vi "MercuryIPSWait.vi"(0 "Inst_param":T3={"Kind"=0, "Strings"=["", "192.168.137.3", "T", "GRPZ"], "uint64s"=[], "Doubles"=[-12.0, 12.0, 6.285], "DAQmx take out list"=[]}) -> ()   [LabVIEW 2013]
uses:
  <instrlib>/Mercury iXX/Public/Controls/Comms Transport Layer.ctl
  <instrlib>/Mercury iXX/Public/Controls/Serial Settings.ctl
  <instrlib>/Mercury iXX/Public/Controls/ISOBus Address.ctl
  <instrlib>/Mercury iXX/Mercury iXX.lvlib
panel:
  out "Mag_data":T1
  out "Device Details":T2={"Devices"=["DB3.L1:LVL", "GRPS:PSU", "GRPX:PSU", "GRPY:PSU", "GRPZ:PSU", "MB1.T1:TEMP", "PSU.M1:PSU", "PSU.M2:PSU"], "S/W Version(s)"=[], "Serial Number(s)"=[]}
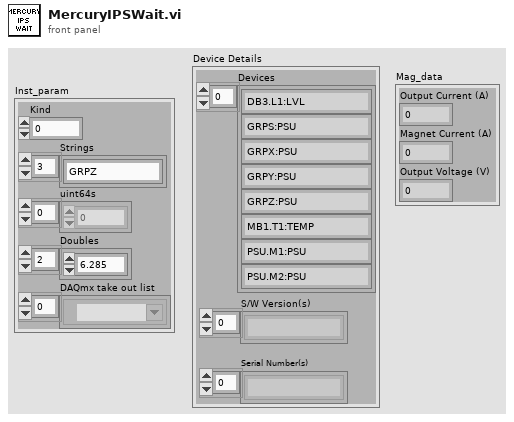
[diagram p1: front panel]
types:
  T1 = cluster{"Output Current (A)":dbl, "Magnet Current (A)":dbl, "Output Voltage (V)":dbl}
  T2 = cluster{"Devices":string[], "S/W Version(s)":string[], "Serial Number(s)":string[]}
  T3 = cluster{"Kind":u16, "Strings":string[], "uint64s":u64[], "Doubles":dbl[], "DAQmx take out list":refnum<k21>[]}
  T4 = typedef "Mercury iXX.lvlib/Comms Transport Layer.ctl" = enum16{"Ethernet TCP/IP", "USB", "ISOBus - RS-232", "GPIB"}
  T5 = typedef "Mercury iXX.lvlib/Serial Settings.ctl" = cluster{"Baud Rate":u32, "Parity":u16, "Data Bits":u16, "Stop Bits":u16, "Flow Control":u16}
  T6 = typedef "Mercury iXX.lvlib/ISOBus Address.ctl" = i32
  T7 = cluster{"VISA resource name":refnum<visa-resource-name>, "Comms Layer":T4, "IP Address":string, "Serial Configuration":T5, "ISOBUS address":T6}
  T8 = typedef "Mercury iXX.lvlib/Mercury Reference.ctl" = cluster{"Comms":refnum<visa-resource-name>, "Device ID":string[], "Comms Layer":T4, "Command":string, "Query reference":T9}
  T9 = typedef "Mercury iXX.lvlib/Query Dynamic Reference.ctl" = refnum<vi>
  T10 = enum16{"Monitor", "Hold", "Clamp", "To Set", "To Zero", "Switch Heater", "Set Points"}
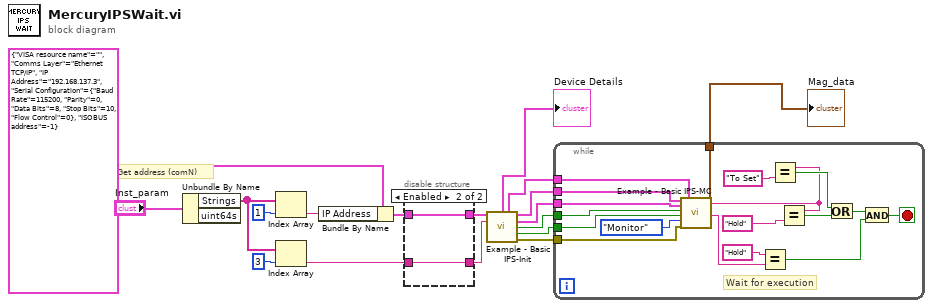
[diagram p0: block diagram]
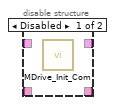
[diagram p2: hidden frame]
diagram:
  # "Get address (comN)"
  n1 = Unbundle By Name("Inst_param") -> ("Strings"=w4:string[])  [unwired: 1 out]
  n2 = Index Array(array=w4, index=1) -> (element=w17:string)
  n3 = Index Array(array=w4, index=3) -> (element=w2:string)
  n4 = Bundle By Name(cluster=T7 {"VISA resource name"="", "Comms Layer"=enum."Ethernet TCP/IP", "IP Address"="192.168.137.3", "Serial Configuration"={"Baud Rate"=115200, "Parity"=0, "Data Bits"=8, "Stop Bits"=10, "Flow Control"=0}, "ISOBUS address"=-1} ("Connection Details"), "IP Address"=w17) -> (w15:T7)
  n5 = disable-structure shown="Enabled" {
    disable-tunnel: [_ w20] -> w13
    disable-tunnel: w15 -> [_ w20]
    disable-tunnel: [_ w19] -> w3
    disable-tunnel: w2 -> [_ w19]
    frame Disabled {
      n6 = call "MDrive_Init_Com.vi"() -> ()  [unwired: 7 in, 2 out]
    }
    frame Enabled {
    }
  }
  n7 = call <instrlib>:"Example - Basic IPS-Init.vi"("Connection Details"=w13, "Axis Group"=w3) -> ("Device Details"=→"Device Details":T2, "Merc_Ref_LVL"=w8:T8, "Merc_Ref_Mag"=w9:T8, "Merc_Ref_MB1.T1"=w7:T8, "Temp_Present?"=w12:bool, "LVL_Present?"=w11:bool, "error out"=w10:errorcluster)  [unwired: 4 in, 3 out]
  n8 = while {
    tunnel: w12 -> [w37]
    tunnel: w11 -> [w36]
    tunnel: w10 -> [w35]
    tunnel: w9 -> [w34]
    tunnel: w8 -> [w33]
    tunnel: w7 -> [w32]
    tunnel: [w21] -> w1
    stop <- w24 stop-if-true
    # "Wait for execution"
    n9 = call <instrlib>:"Example - Basic IPS-MC.vi"("Mag_Ref"=w34, "MB1.T1_Ref"=w32, "Temp_present?"=w37, "LVL_present?"=w36, "Action"=T10."Monitor", "error in (no error)"=w35, "LVL_Ref"=w33) -> ("Mag_data"=w21:T1, "Status"=w25:string, "Mode"=w30:string)  [unwired: 7 in, 3 out]
    n10 = Equal?(x="Hold", y=w30) -> (x = y?=w23:bool)
    n11 = Equal?(x=w25, y="To Set") -> (x = y?=w27:bool)
    n12 = Equal?(x=w25, y="Hold") -> (x = y?=w26:bool)
    n13 = Or(x=w27, y=w26) -> (x .or. y?=w22:bool)
    n14 = And(x=w22, y=w23) -> (x .and. y?=w24:bool)
  }
  "Mag_data" <- w1
